vi "FindProjectPath.vi"(8 "error in (no error)":errorcluster, 11 "Library Name":string) -> (0 "error out":errorcluster, 2 "Found?":bool, 3 "Project Path":path)   [LabVIEW 2023, in "CICD.lvlib"]
uses:
  CICD.lvlib
  <userlib>/_OpenG.lib/file/file.llb/openg_file.lvlib
  <vilib>/SLL Toolkit/SLL String/SLL String.lvlib
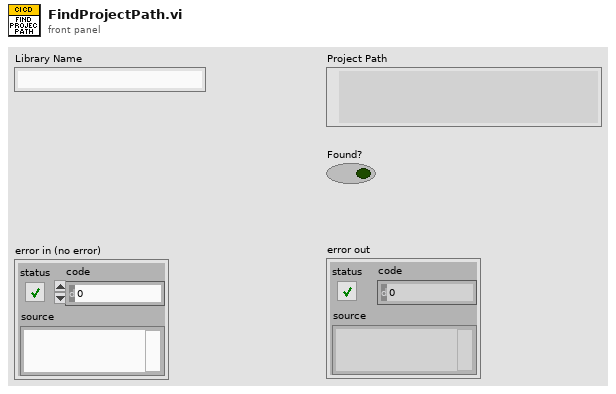
[diagram p1: front panel]
types:
  T1 = typedef "CICD.lvlib/CICDPathConfigs.ctl" = cluster{"GlobalIncludePaths":path[], "GlobalExcludePaths":path[], "BuildSpecsIncludePaths":path[], "ActualDepsIncludePaths":path[], "WorkspacePath":path, "SourceFolderPaths":path[], "ChangedFilesLogpaths":map{string, path}}
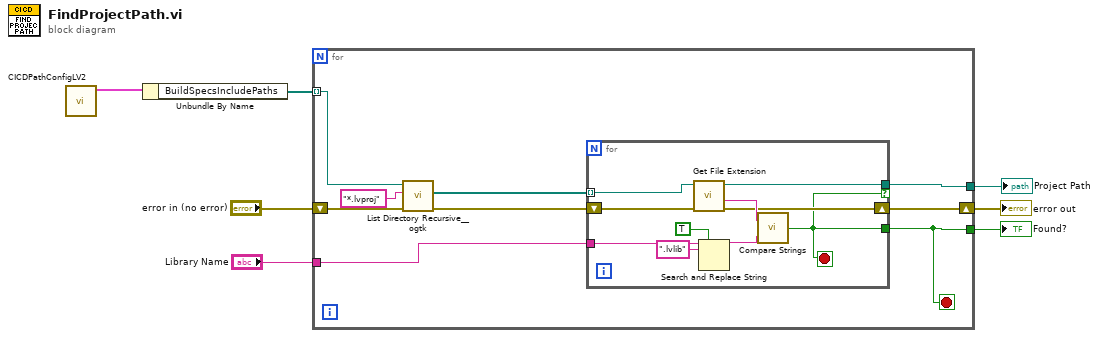
[diagram p0: block diagram]
diagram:
  n1 = call "CICDPathConfigLV2.vi"() -> ("CICD Path Config Out"=w2:T1)  [unwired: 11 in]
  n2 = Unbundle By Name(w2) -> ("BuildSpecsIncludePaths"=w1:path[])
  n3 = for {
    tunnel: [w15] -> w6
    tunnel: [w8] -> w5
    tunnel: "Library Name" -> [w13]
    shift-right: [w10] -> w3
    shift-left: "error in (no error)" -> [w16]
    tunnel: w1 -> [w9] mode=indexing
    stop <- w8 stop-if-true
    n4 = call <userlib>:"List Directory Recursive__ogtk.vi"("error in (no error)"=w16, "pattern"="*.lvproj", "Path"=w9) -> ("error out"=w14:errorcluster, "file paths"=w12:path[])  [unwired: 5 in, 2 out]
    n5 = for {
      tunnel: w12 -> [w25] mode=indexing
      tunnel: w13 -> [w24]
      shift-right: [w19] -> w10
      shift-left: w14 -> [w26]
      tunnel: [w18] -> w15 if=w17
      tunnel: [w17] -> w8
      stop <- w17 stop-if-true
      n6 = call <vilib>:"Get File Extension.vi"("error in (no error)"=w26, "file"=w25) -> ("error out"=w19:errorcluster, "filename without extension"=w21:string, "dup file"=w18:path)  [unwired: 5 in, 2 out]
      n7 = Search and Replace String(replace all?=TRUE ("replace all? (F)"), input string=w24, search string=".lvlib") -> (result string=w20:string)  [unwired: 5 in, 3 out]
      n8 = call <vilib>:"Compare Strings.vi"("y"=w20, "x"=w21) -> ("Equal?"=w17:bool)
    }
  }
  "Project Path" <- w6
  "Found?" <- w5
  "error out" <- w3
